vi "write exit message.vi"() -> (2 "queue out":refnum<queue>, 3 "message":refnum<class "communicator message.lvclass">)   [LabVIEW 2015, in "communicator.lvclass"]
uses:
  communicator.lvclass
  message/communicator message.lvclass
  message/communicator message.lvclass/communicator message.ctl
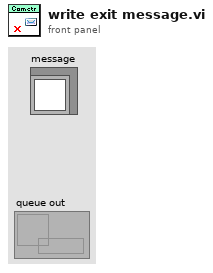
[diagram p1: front panel]
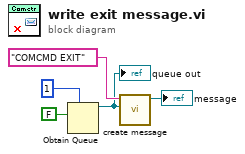
[diagram p0: block diagram]
diagram:
  n1 = Obtain Queue(max queue size (-1, unlimited)=1, element data type=FALSE) -> (queue out=w2:refnum<queue>)  [unwired: 3 in, 2 out]
  "queue out" <- w2
  n2 = call "create message.vi"("data"=w2, "ID"="COMCMD EXIT") -> ("message"=→"message":refnum<class "communicator message.lvclass">)  [unwired: 9 in]
